vi "Write ErrorData.vi"(8 "error in (no error)":errorcluster, 10 "ErrorData":T2, 11 "Error in":refnum<class "Error.lvclass">) -> (0 "error out":errorcluster, 3 "Error out":refnum<class "Error.lvclass">)   [LabVIEW 2019, in "Error.lvclass"]
uses:
  Error.lvclass
  TypeDef/Error Classification.ctl
  Error.lvclass/Error.ctl
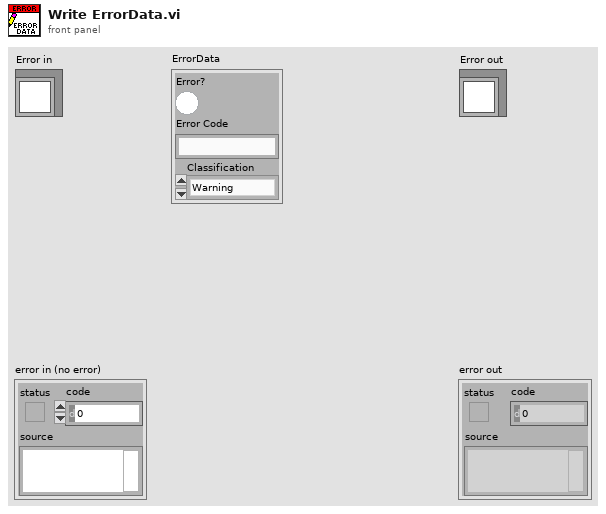
[diagram p1: front panel]
types:
  T1 = typedef "Error.lvclass/Error Classification.ctl" = enum16{"Warning"}
  T2 = cluster{"Error?":bool, "Error Code":string, "Classification":T1}
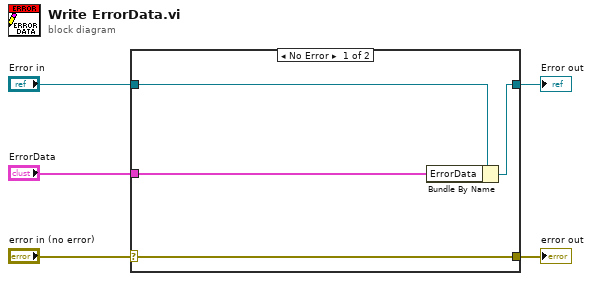
[diagram p0: block diagram]
diagram:
  n1 = case shown="No Error" "error in (no error)" {
    selector: "error in (no error)" -> [w9 w10]
    tunnel: [w9 w10] -> w4
    tunnel: [w7 w11] -> w2
    tunnel: "Error in" -> [w8 w11]
    tunnel: "ErrorData" -> [w6 _]
    frame No Error {
      n2 = Bundle By Name(cluster=w8, "ErrorData"=w6) -> (w7:refnum<class "Error.lvclass">)
    }
    frame Error {
    }
  }
  "error out" <- w4
  "Error out" <- w2
